vi "fpga_RefCH Process (M Class_50Hz).vi"(0 "data in <?24.1>":fxp<+/-,24,1>, 1 "Memory In":refnum<k21>="coefROM", 5 "Channel number":u8, 7 "Reference index":u8, 9 "input data valid":bool, 12 "ready for output":bool) -> (4 "Filtered Ref data":fxp<+/-,24,3> format="%.22g", 10 "output valid":bool, 14 "ready for input":bool, 15 "error":i32)   [LabVIEW 2013, in "NI_EP_PMU_FPGA.lvlib"]
uses:
  <vilib>/addons/Electrical Power/PMU/NI_EP_PMU_FPGA.lvlib
  <vilib>/rvi/FXPMathLib/basic elements/FxpDiscreteDelay/XNode/nifxpmath_DiscreteDelay.xnode
  <vilib>/addons/Electrical Power/PQ/Resampling/NI_EP_Resample_FPGA.lvlib
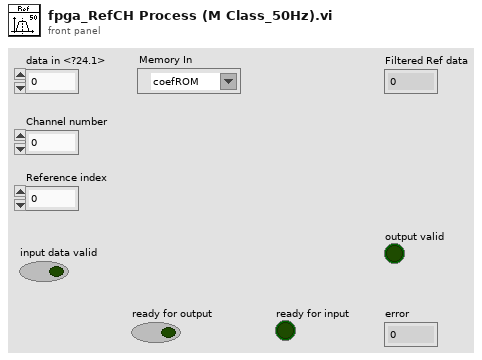
[diagram p1: front panel]
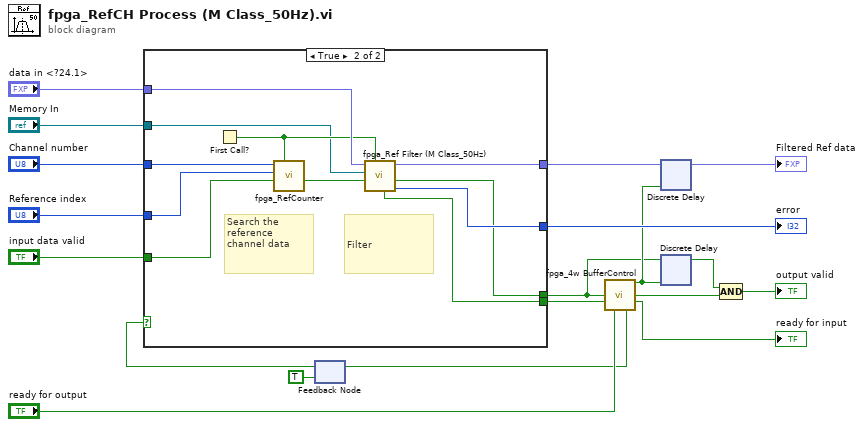
[diagram p0: block diagram]
diagram:
  n1 = feedback #1(TRUE ("ready for output")) -> (w10:bool)
  n2 = case shown="True" w10 {
    tunnel: "input data valid" -> [_ w30]
    tunnel: "Reference index" -> [_ w29]
    tunnel: "Channel number" -> [_ w28]
    tunnel: "data in <?24.1>" -> [_ w27]
    tunnel: "Memory In" -> [_ w24]
    tunnel: [_ w23] -> w14
    tunnel: [_ w22] -> w8
    tunnel: [_ w21] -> w5
    tunnel: [_ w20] -> w13
    frame False {
    }
    frame True {
      # "Filter"
      # "Search the reference channel data"
      n3 = First Call?() -> (First Call?: T/F=w25:bool)
      n4 = call <vilib>:"fpga_RefCounter.vi"("reset"=w25, "input valid?"=w30, "Reference index"=w29, "NChan"=w28) -> ("Reference channel input valid"=w26:bool)  [unwired: 6 in, 1 out]
      n5 = call <vilib>:"fpga_Ref Filter (M Class_50Hz).vi"("reset"=w25, "input valid"=w26, "Memory In"=w24, "input data"=w27) -> ("error"=w23:i32, "output valid"=w21:bool, "output data <i24,3>"=w22:fxp<+/-,24,3>, "ready for input"=w20:bool)  [unwired: 4 in]
    }
  }
  "error" <- w14
  n6 = call <vilib>:"fpga_4w BufferControl.vi"("DR"=w5, "RFI"=w13, "RFO"="ready for output") -> ("buff enable"=w6:bool, "output valid"=w4:bool, "ready for input"=→"ready for input":bool, "logic enable"=w9:bool)  [unwired: 9 in]
  n7 = feedback-in #1(w9) -> ()
  n8 = xnode ("Discrete Delay")("D"=w8, "enable"=w6) -> ("Q"=→"Filtered Ref data":fxp<+/-,24,3>)
  n9 = xnode ("Discrete Delay")("D"=w5, "enable"=w6) -> ("Q"=w3:bool)
  n10 = Compound Arithmetic op=AND(w3, w4) -> (→"output valid":bool)
